vi "Server Status.vi"(8 "error in (no error)":errorcluster, 11 ".NET Refnum in":refnum<k24>) -> (0 "error out":errorcluster, 3 "Cluster":T1)   [LabVIEW 2024, in "LV_OPC_NET.lvlib"]
uses:
  LV_OPC_NET.lvlib
  C:/Users/108003658/OneDrive - Baker Hughes/Desktop/LV_OPC-Client-x64/LV_OPC_Test/OPC.NET/OpcNetApi.dll
  OpcNetApi.dll
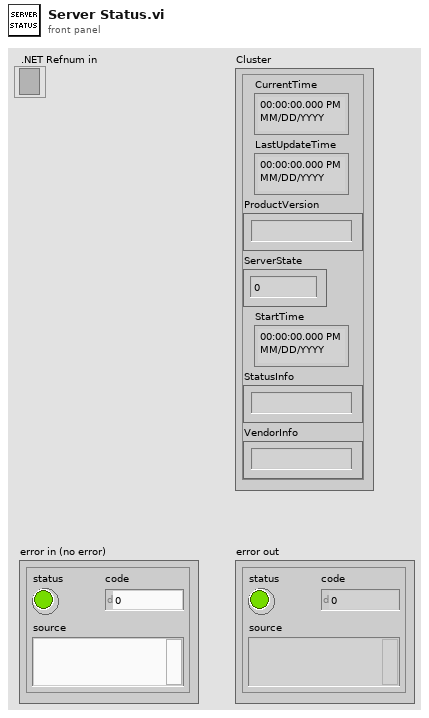
[diagram p1: front panel]
types:
  T1 = cluster{"CurrentTime":timestamp, "LastUpdateTime":timestamp, "ProductVersion":string, "ServerState":i32, "StartTime":timestamp, "StatusInfo":string, "VendorInfo":string}
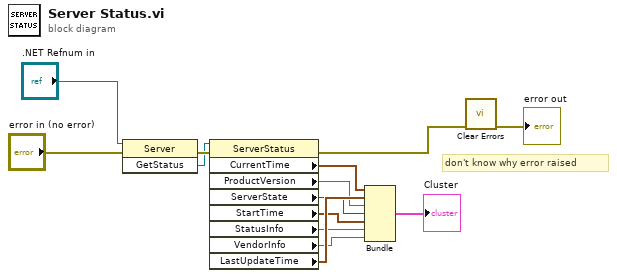
[diagram p0: block diagram]
diagram:
  # "don't know why error raised"
  n1 = invoke class="Server" method="GetStatus"(reference=".NET Refnum in", error in="error in (no error)") -> (error out=w14:errorcluster, "GetStatus"=w3:refnum<k24>)  [unwired: 1 in, 1 out]
  n2 = property class="ServerStatus"(reference=w3, error in=w14) -> (error out=w12:errorcluster, "CurrentTime"=w4:timestamp, "ProductVersion"=w5:string, "ServerState"=w6:i32, "StartTime"=w7:timestamp, "StatusInfo"=w8:string, "VendorInfo"=w9:string, "LastUpdateTime"=w10:timestamp)  [unwired: 1 out]
  n3 = Bundle("CurrentTime"=w4, "LastUpdateTime"=w10, "ProductVersion"=w5, "ServerState"=w6, "StartTime"=w7, "StatusInfo"=w8, "VendorInfo"=w9) -> (→"Cluster":T1)  [unwired: 1 in]
  n4 = call <vilib>:"Clear Errors.vi"("error in (no error)"=w12) -> ("error out"=→"error out":errorcluster)  [unwired: 5 in, 1 out]
